vi "main.vi"() -> ()   [LabVIEW 2013]
panel:
  out "Index":i32
  out "Number of Particles":i32
  out "Time(s)":i32
  out "XY Graph":cluster{u32[], i32[]}(graph)
  in  "End Index":i32=1700
  in  "Start Index":i32=1500
  in  "File Name":string="cameraA-nr"
  out "Image Out":T1(plugin-control)
  out "Particle Measurements (Pixels)":dbl[][](array[numeric]) format="%.2f"
  out "error out":errorcluster
  in  "error in":errorcluster
  in  "Path":path=path "Z:/Downloads/Fridge Pictures/1"
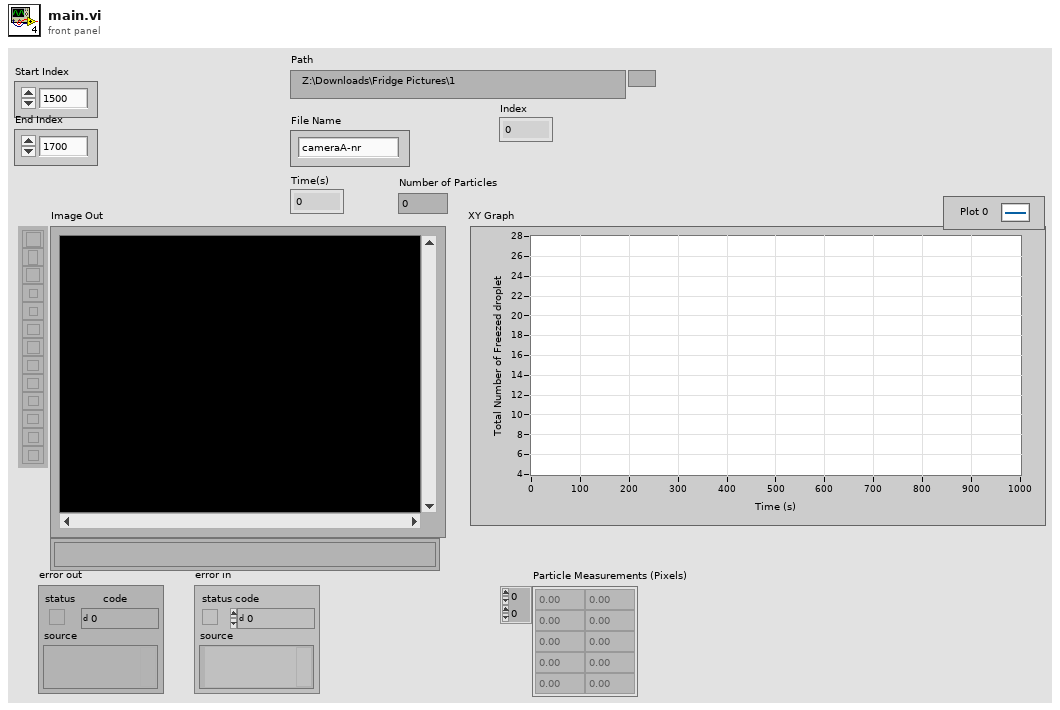
[diagram p1: front panel]
types:
  T1 = typedef "IMAQ Image.ctl" = refnum<image>
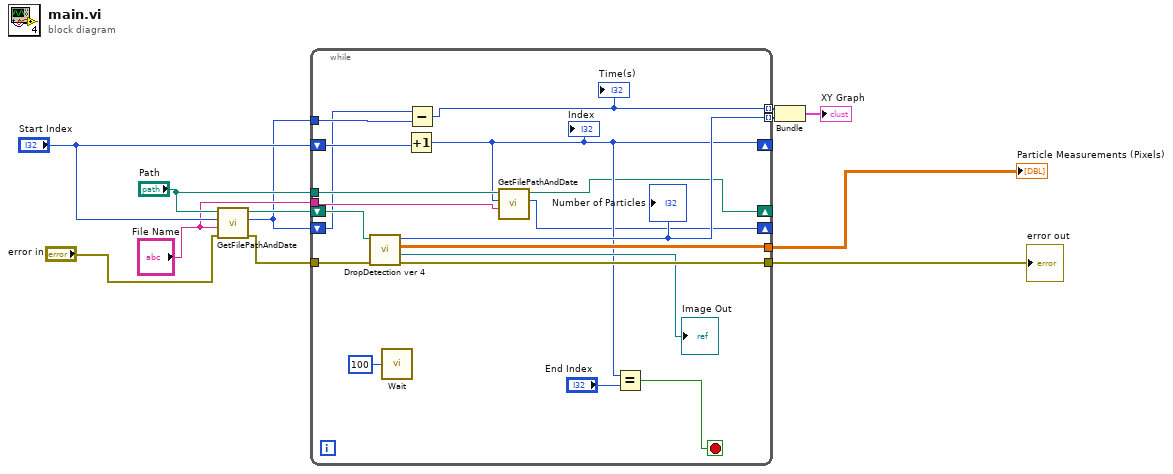
[diagram p0: block diagram]
diagram:
  n1 = call "GetFilePathAndDate.vi"("error in (no error)"="error in", "String"="File Name", "Index"="Start Index", "Path"="Path") -> ("error out"=w5:errorcluster, "creation date"=w1:u32, "file out"=w4:path)  [unwired: 5 in]
  n2 = while {
    tunnel: w5 -> [w30]
    tunnel: [w29] -> w12
    tunnel: [w28] -> w9 mode=indexing
    tunnel: [w27] -> w11
    shift-right: [w18] -> _
    shift-left: "Start Index" -> [w24]
    tunnel: [w23] -> w10 mode=indexing
    tunnel: "Path" -> [w20]
    tunnel: "File Name" -> [w19]
    shift-right: [w17] -> _
    shift-left: w4 -> [w21]
    shift-right: [w16] -> _
    shift-left: w1 -> [w14]
    tunnel: w1 -> [w15]
    stop <- w25 stop-if-true
    n3 = call "DropDetection ver 4.vi"("error in"=w30, "Path"=w21) -> ("error out"=w29:errorcluster, "Image Out"=→"Image Out":T1, "Particle Measurements (Pixels)"=w27:dbl[][], "Number of Particles"=w28:i32)  [unwired: 6 in]
    "Number of Particles" <- w28
    n4 = call "Wait"("Count(mSec)"=u32 100) -> ()  [unwired: 1 out]
    n5 = Increment(x=w24) -> (x+1=w18:i32)
    "Index" <- w18
    n6 = Subtract(x=w14, y=w15) -> (x-y=w23:u32)
    "Time(s)" <- w23
    n7 = call "GetFilePathAndDate.vi"("String"=w19, "Index"=w18, "Path"=w20) -> ("creation date"=w16:u32, "file out"=w17:path)  [unwired: 6 in, 1 out]
    n8 = Equal?(x=w18, y="End Index") -> (x = y?=w25:bool)
  }
  "error out" <- w12
  "Particle Measurements (Pixels)" <- w11
  n9 = Bundle(w10, w9) -> (→"XY Graph":cluster{u32[], i32[]})  [unwired: 1 in]
